vi "subExpandExternalDepsInLocation.vi"(8 "error in (no error)":errorcluster, 11 "SolutionBuilder in":refnum<class "SolutionBuilder.lvclass">) -> (0 "error out":errorcluster, 3 "SolutionBuilder out":refnum<class "SolutionBuilder.lvclass">)   [LabVIEW 2019, in "SolutionBuilder.lvlib" / "SolutionBuilder.lvclass"]
uses:
  SolutionBuilder.lvclass
  <vilib>/Utility/miscctls.llb/LVMapReplaceAction.ctl
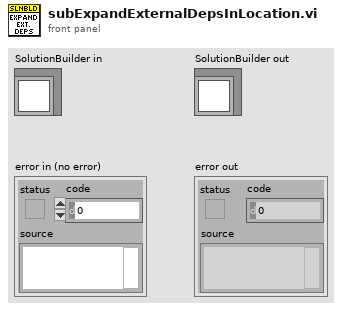
[diagram p1: front panel]
types:
  T1 = typedef "LVMapReplaceAction.ctl" = enum32{"Modify Entry only if found", "Add or Modify Entry", "Delete Entry"}
  T2 = typedef "SolutionBuilder.lvlib/SolutionBuilder.lvclass/ProjectItemMap.ctl" = map{path, refnum<class "ProjectItem.lvclass">[]}
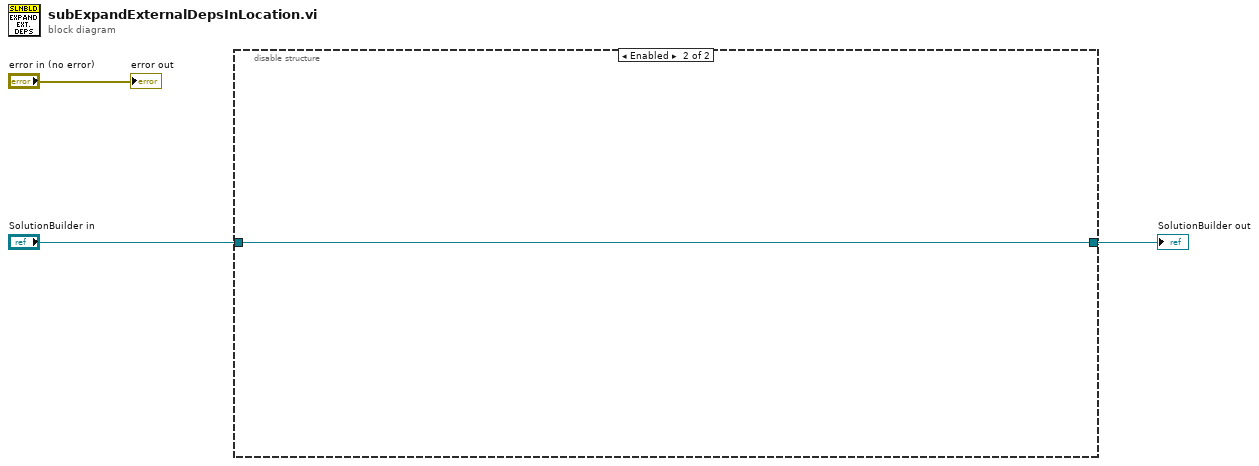
[diagram p0: block diagram]
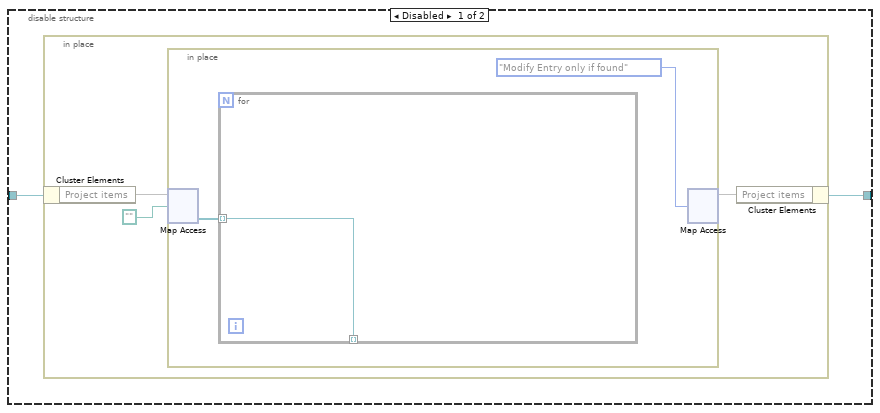
[diagram p2: hidden frame]
diagram:
  n1 = disable-structure shown="Enabled" {
    disable-tunnel: "SolutionBuilder in" -> [w5 w12]
    disable-tunnel: [w4 w12] -> w1
    frame Disabled {
      n2 = in-place {
        n3 = in-place-cluster #1(w5) -> ("Project items"=w8:T2)
        n4 = in-place {
          n5 = in-place-map #2(w8, path "") -> (w9:refnum<class "ProjectItem.lvclass">[])  [unwired: 1 in, 1 out]
          n6 = for {
            tunnel: w9 -> [w11] mode=indexing
            tunnel: [w11] -> _ mode=indexing
          }
          n7 = in-place-map #2(LVMapReplaceAction."Modify Entry only if found" ("action")) -> (w7:T2)  [unwired: 1 in, 2 out]
        }
        n8 = in-place-cluster #1("Project items"=w7) -> (w4:refnum<class "SolutionBuilder.lvclass">)
      }
    }
    frame Enabled {
    }
  }
  "SolutionBuilder out" <- w1
  "error out" <- "error in (no error)"
